vi "AoC21-Read bingo input file.vi"(11 "input file":path) -> (1 "Bingo Cards":i32[][][](array[numeric]), 2 "input text":string, 3 "bingo calls":i32[](array[numeric]))   [LabVIEW 2021]
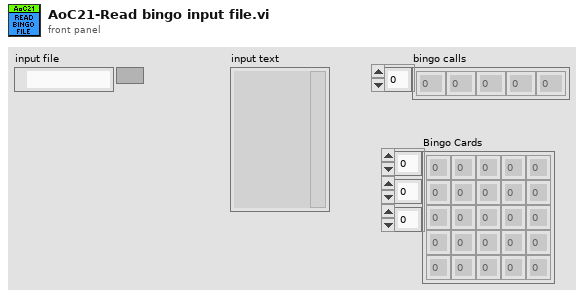
[diagram p1: front panel]
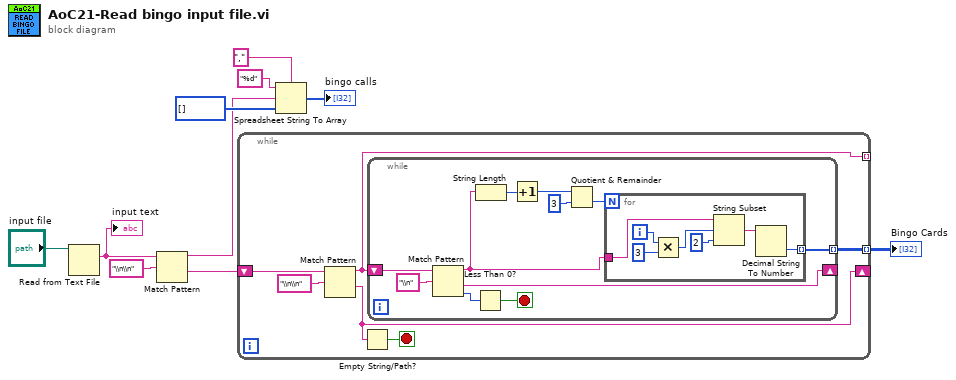
[diagram p0: block diagram]
diagram:
  n1 = Read from Text File(file (use dialog)="input file") -> (text=w6:string)  [unwired: 3 in, 3 out]
  "input text" <- w6
  n2 = Match Pattern(string=w6, regular expression="\\n\\n") -> (before substring=w4:string, after substring=w2:string)  [unwired: 1 in, 2 out]
  n3 = while {
    shift-right: [w14] -> _
    shift-left: w2 -> [w15]
    tunnel: [w12] -> w1 mode=indexing
    tunnel: [w11] -> _ mode=indexing
    stop <- w13 stop-if-true
    n4 = Match Pattern(string=w15, regular expression="\\n\\n") -> (before substring=w11:string, after substring=w14:string)  [unwired: 1 in, 2 out]
    n5 = Empty String/Path?(string/path=w14) -> (empty?=w13:bool)
    n6 = while {
      shift-right: [w25] -> _
      shift-left: w11 -> [w27]
      tunnel: [w22] -> w12 mode=indexing
      stop <- w23 stop-if-true
      n7 = Match Pattern(string=w27, regular expression="\\n") -> (before substring=w21:string, after substring=w25:string, offset past match=w24:i32)  [unwired: 1 in, 1 out]
      n8 = Less Than 0?(x=w24) -> (x < 0?=w23:bool)
      n9 = String Length(string=w21) -> (length=w20:i32)
      n10 = Increment(x=w20) -> (x+1=w19:i32)
      n11 = Quotient & Remainder(x=w19, y=3) -> (floor(x/y)=w17:i32)  [unwired: 1 out]
      n12 = for {
        N: w17 -> [_]
        tunnel: [w28] -> w22 mode=indexing
        tunnel: w21 -> [w30]
        i -> [w34]
        n13 = Multiply(x=w34, y=3) -> (x*y=w32:i32)
        n14 = String Subset(string=w30, offset (0)=w32, length (rest)=2 ("length (rest)")) -> (substring=w29:string)
        n15 = Decimal String To Number(string=w29) -> (number=w28:i32)  [unwired: 2 in, 1 out]
      }
    }
  }
  "Bingo Cards" <- w1
  n16 = Spreadsheet String To Array(delimiter (Tab)=",", format string="%d", spreadsheet string=w4, array type (2D Dbl)=i32[] []) -> (array=→"bingo calls":i32[])
